vi "Change Setting.vi"(8 "error in (no error)":errorcluster, 10 "Change setting mode":T1=enum."Next", 11 "Device in":refnum<class "CK.lvclass">) -> (0 "error out":errorcluster, 1 "Changes":cluster{"Name":string, "Value":string}[](array[cluster]), 2 "Last setting":bool, 3 "Device out":refnum<class "CK.lvclass">)   [LabVIEW 2020, in "CK.lvclass"]
uses:
  CK.lvclass
  Controls/Change setting mode enum.ctl
  PIC-device/PIC-Device.lvclass
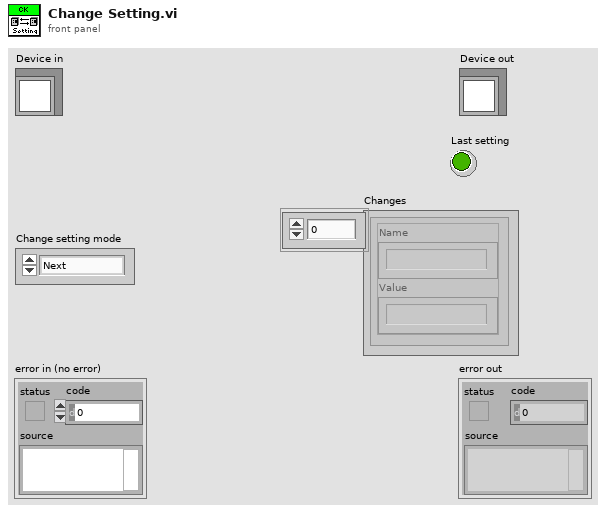
[diagram p1: front panel]
types:
  T1 = typedef "PIC-Device.lvclass/Change setting mode enum.ctl" = enum16{"Init", "Next", "Reset"}
  T2 = typedef "PIC-Device.lvclass/Register to Write.ctl" = cluster{"Register":u32, "Value":u32, "Dev Address":u32, "Physical Adress":u32}
  T3 = cluster{"Cap states reg":T2[], "Cap states":dbl[], "Cap sweep string":string}[]
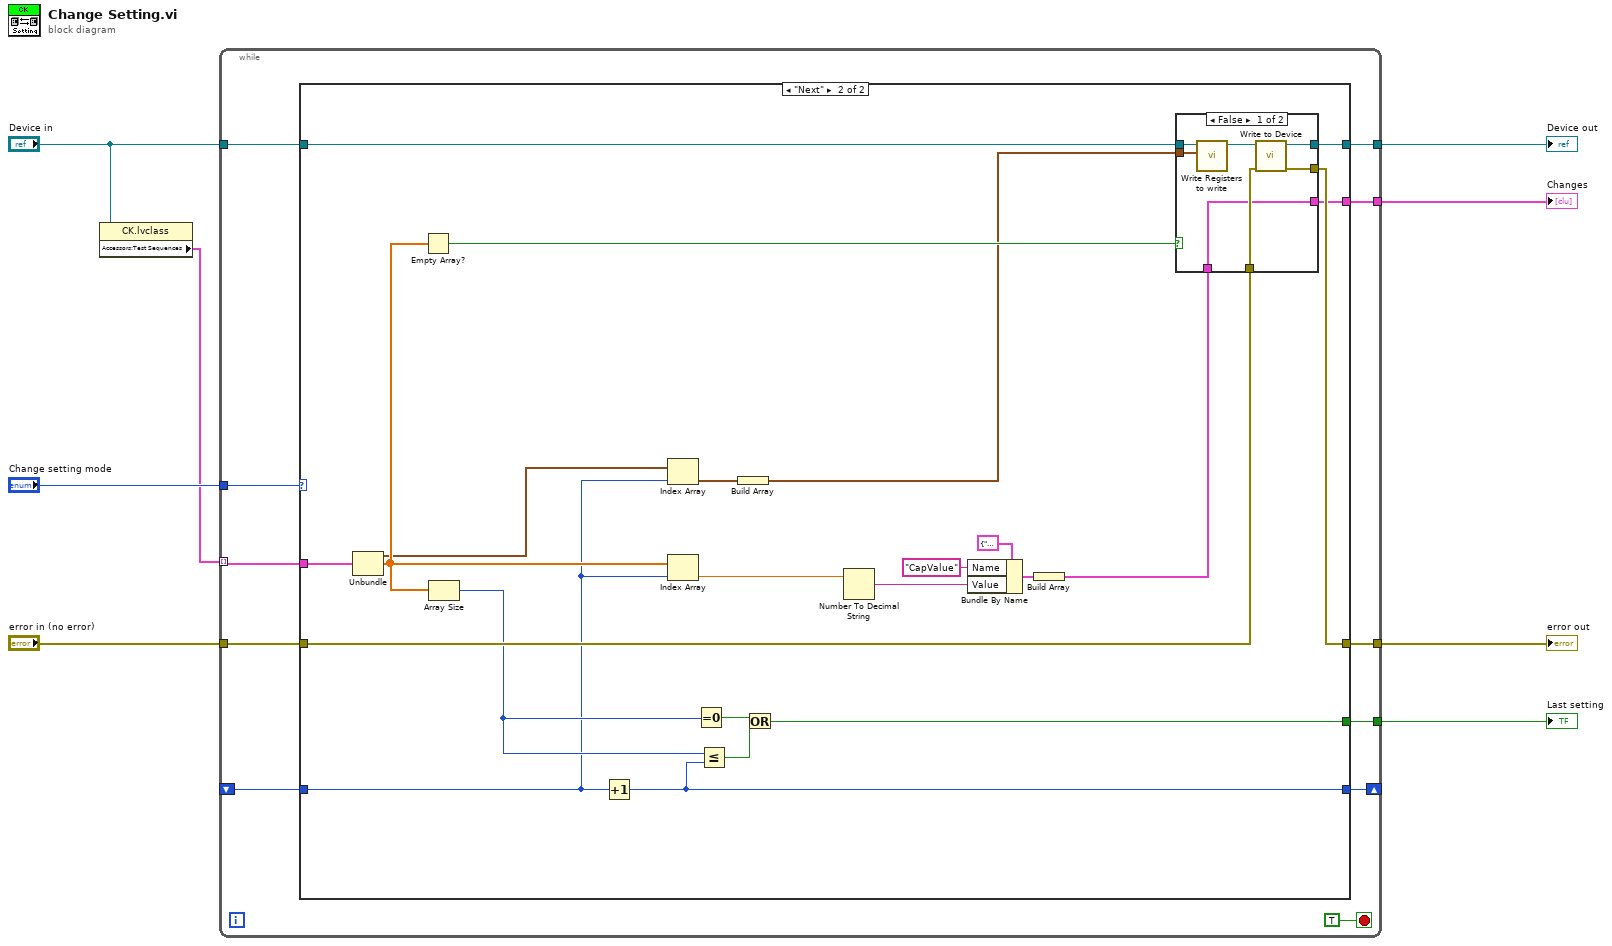
[diagram p0: block diagram]
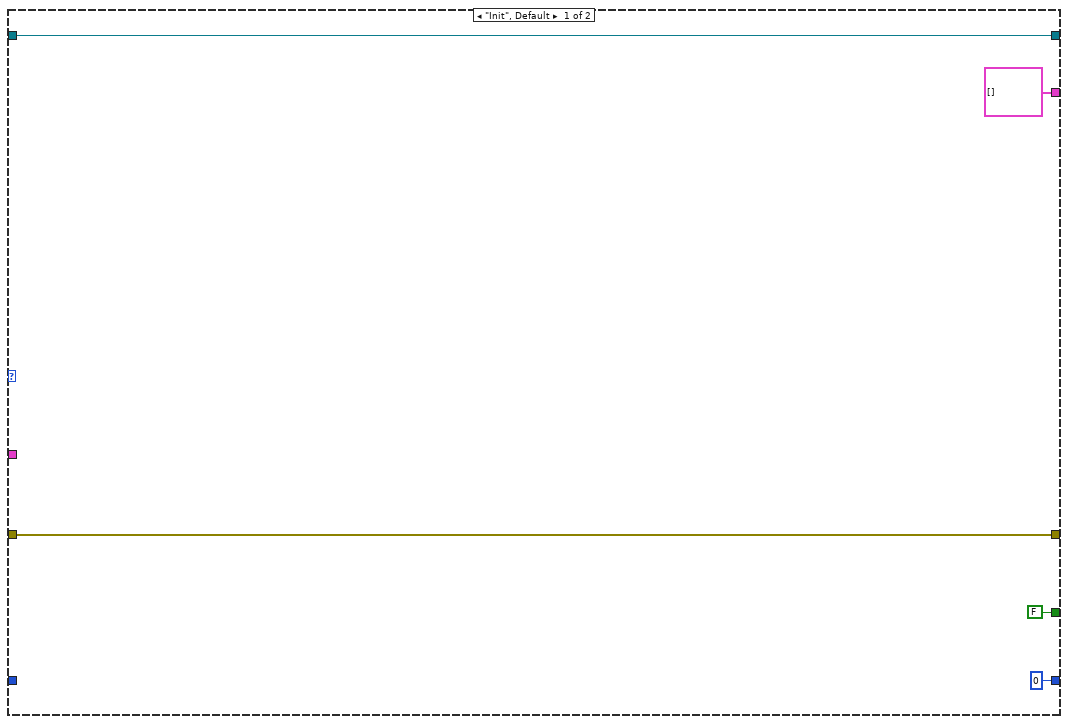
[diagram p2: hidden frame]
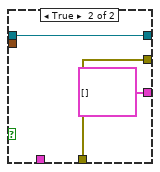
[diagram p3: hidden frame]
diagram:
  n1 = property class="CK.lvclass"(reference="Device in") -> ("Accessors:Test Sequences"=w1:T3)  [unwired: 1 in, 2 out]
  n2 = while {
    tunnel: w1 -> [w19] mode=indexing
    tunnel: "Change setting mode" -> [w17]
    shift-right: [w16] -> _
    shift-left: _ -> [w15]
    tunnel: "Device in" -> [w14]
    tunnel: [w13] -> w4
    tunnel: [w12] -> w5
    tunnel: "error in (no error)" -> [w11]
    tunnel: [w10] -> w7
    tunnel: [w9] -> w6
    stop <- TRUE stop-if-true
    n3 = case shown="\"Next\"" w17 {
      tunnel: w19 -> [_ w47]
      tunnel: [0 w43] -> w16
      tunnel: w15 -> [_ w25]
      tunnel: w14 -> [w20 w45]
      tunnel: [w20 w44] -> w13
      tunnel: [FALSE w37] -> w12
      tunnel: w11 -> [w22 w42]
      tunnel: [w22 w41] -> w10
      tunnel: [cluster{"Name":string, "Value":string}[] [] w40] -> w9
      frame "Init", Default {
      }
      frame "Next" {
        n4 = Unbundle(w47) -> ("Cap states reg"=w28:T2[], "Cap states"=w30:dbl[])  [unwired: 1 out]
        n5 = Empty Array?(array=w30) -> (empty?=w46:bool)
        n6 = Array Size(array=w30) -> (size(s)=w29:i32)
        n7 = Increment(x=w25) -> (x+1=w43:i32)
        n8 = Index Array(array=w28, index=w25) -> (element=w27:T2)
        n9 = Index Array(array=w30, index=w25) -> (element=w35:dbl)
        n10 = Equal To 0?(x=w29) -> (x = 0?=w39:bool)
        n11 = Less Or Equal?(x=w29, y=w43) -> (x <= y?=w38:bool)
        n12 = Build Array(w27) -> (w26:T2[])
        n13 = Or(x=w39, y=w38) -> (x .or. y?=w37:bool)
        n14 = Number To Decimal String(number=w35) -> (decimal integer string=w31:string)  [unwired: 1 in]
        n15 = Bundle By Name(cluster=cluster{"Name":string, "Value":string} {"Name"="", "Value"=""} ("Change"), "Name"="CapValue", "Value"=w31) -> (w33:cluster{"Name":string, "Value":string})
        n16 = Build Array(w33) -> (w36:cluster{"Name":string, "Value":string}[])
        n17 = case shown="False" w46 {
          tunnel: w45 -> [w54 w57]
          tunnel: w26 -> [w53 _]
          tunnel: [w51 w57] -> w44
          tunnel: [w50 w55] -> w41
          tunnel: [w48 cluster{"Name":string, "Value":string}[] []] -> w40
          tunnel: w42 -> [w49 w55]
          tunnel: w36 -> [w48 _]
          frame False {
            n18 = call-dynamic "Write Registers to write.vi"("Registers to write"=w53, "Device in"=w54) -> ("Device out"=w52:refnum<class "CK.lvclass">)  [unwired: 9 in]
            n19 = call-dynamic "Write to Device.vi"("error in (no error)"=w49, "Device in"=w52) -> ("error out"=w50:errorcluster, "Device out"=w51:refnum<class "CK.lvclass">)  [unwired: 7 in, 1 out]
          }
          frame True {
          }
        }
      }
    }
  }
  "error out" <- w7
  "Device out" <- w4
  "Changes" <- w6
  "Last setting" <- w5
